vi "test Cluster Modify.vi"() -> ()   [LabVIEW 2023]
uses:
  target/debug/liblabview_test_library.dylib
panel:
  out "UserEvent":cluster{"eventno":i32, "id":string}
  out "error out":errorcluster
  out "return type":i32
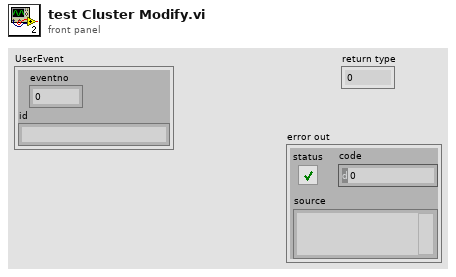
[diagram p1: front panel]
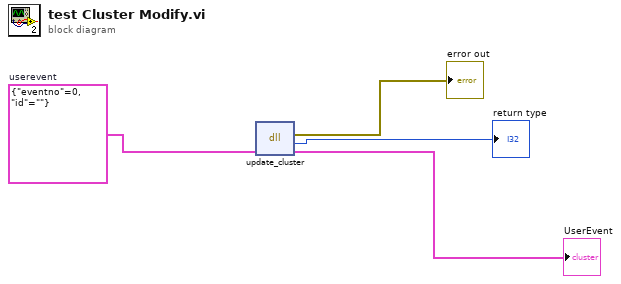
[diagram p0: block diagram]
diagram:
  w2 = cluster{"eventno":i32, "id":string} {"eventno"=0, "id"=""}  # userevent
  n1 = dll-call lib="Volumes/NuFlo/work/src/Rust-LabVIEW-Interop/target/debug/liblabview_test_library.dylib" fn="update_cluster"("UserEvent"=w2) -> (error out=→"error out":errorcluster, "return type"=→"return type":i32, "UserEvent"=→"UserEvent":cluster{"eventno":i32, "id":string})  [unwired: 3 in, 1 out]
